vi "Frequ-sweep.vi"   [LabVIEW 2019]
uses:
  Global/Global Variables/global.vi
  Instrument_Setup.vi
  Global/Global Variables/Data_Display_global.vi
  Monitors/Utility/Monitor Communication/sub-vis/K6221_Open_Queue.vi
types:
  T1 = typedef "15T-Cluster.ctl" = cluster{"Magnet (T)":dbl, "Leads (T)":dbl, "Setpoint (T)":dbl, "Rate (T/min)":dbl, "Set":bool, "Zero":bool, "Hold":bool, "Go to zero":bool, "Go to Hold":bool, "Go to Set":bool, "Clamp":bool, "Switch Heater":bool, "Rate limit":bool, "Switch":bool, "Clamped":bool, "Persistent":bool, "Quenched":bool, "Sweeping":bool, "Select":bool}
  T2 = typedef "PSIO.ctl" = cluster{"Address":T3, "Version":enum16{"PS", "IPS"}}
  T3 = typedef "OxfordAddress.ctl" = cluster{"Com Port":i32, "ISOBUS Address":i32, "GPIB Address":i16, "Communication":enum16{"RS232", "ISOBUS", "GPIB", "Gateway"}}
  T4 = cluster{"Version\n":string, "Max Sweep":dbl[unit], "Max Field":dbl[unit], "IO Info":T2, "Switch htr dly":dbl[unit]}
  T5 = typedef "16T-Cluster.ctl" = cluster{"Clamp":bool, "Switch Heater":bool, "Go to Zero":bool, "Go to set":bool, "Go to Hold":bool, "Clamped":bool, "Quenched":bool, "Rate limit":bool, "Persistent":bool, "Hold":bool, "Set":bool, "Zero":bool, "Magnet (T)":dbl, "Leads (T)":dbl, "Magnet T (K)":dbl, "Switch":bool, "Setpoint (T)":dbl, "Rate (T/min)":dbl, "Select":bool, "Sweeping":bool}
  T6 = cluster{"Version\n":string, "Max Sweep(4.2K)":dbl[unit], "Max Sweep(2.2K)":dbl[unit], "Switch htr dly":dbl[unit], "Max Field(4.2K)":dbl[unit], "Max Field(2.2K)":dbl[unit], "Max lead res":dbl[unit], "IO Info":T2}
  T7 = typedef "K6221_Cluster.ctl" = cluster{"Plot Window":dbl[][], "A":dbl, "A (RMS)":dbl, "Hz":dbl, "I (A)":dbl, "f (Hz)":dbl, "Update":bool, "Offset":dbl, "Offset (A)":dbl, "Compliance":bool, "Output":bool, "Output Status":bool}
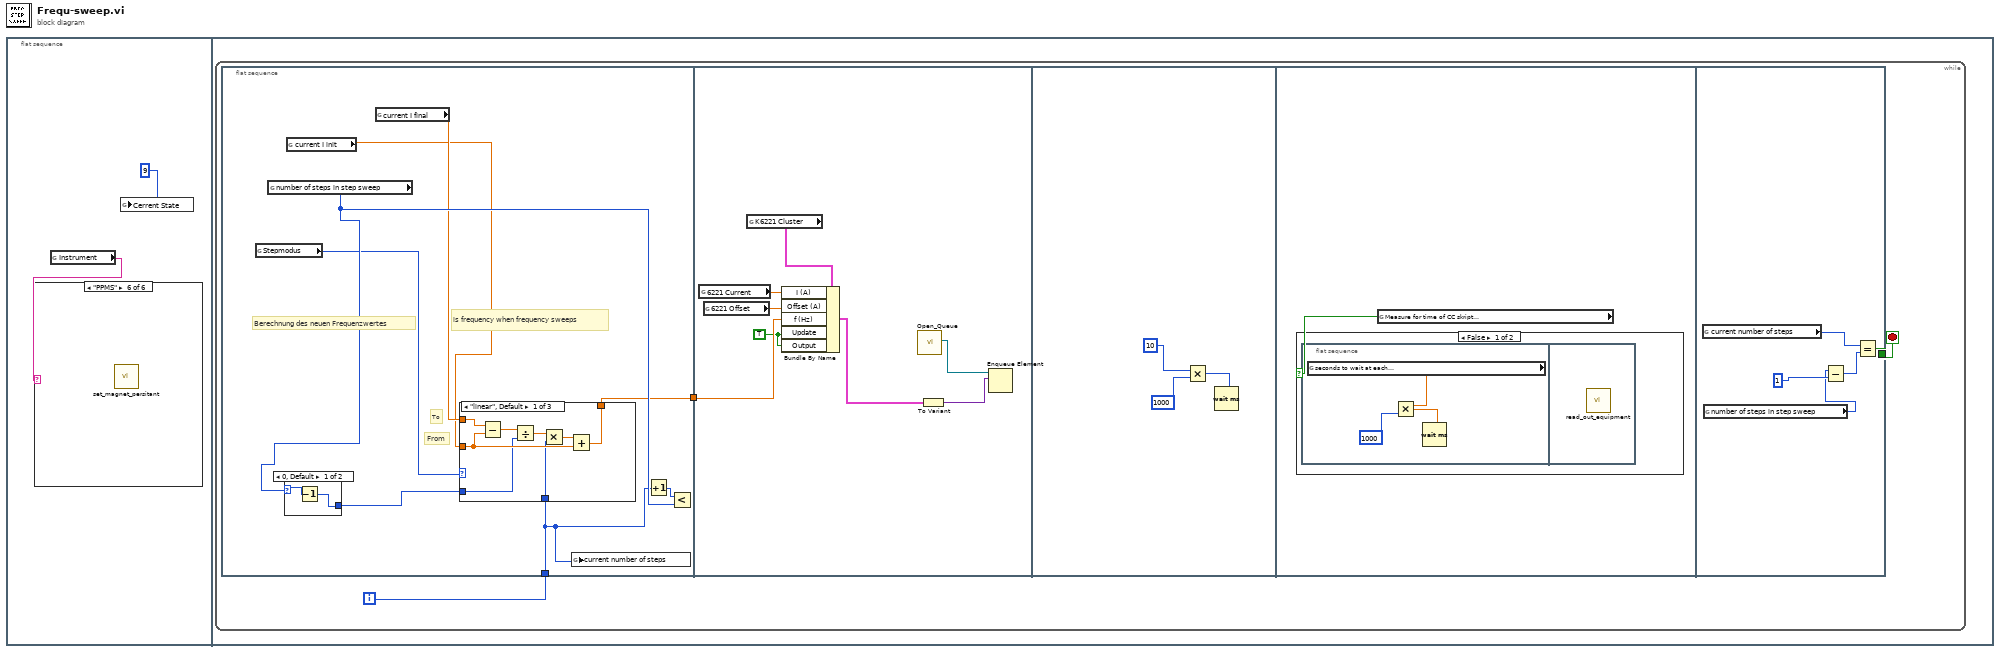
[diagram p0: block diagram]
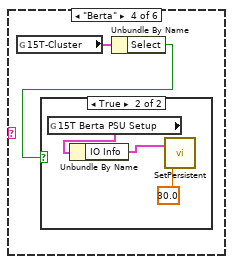
[diagram p5: hidden frame]
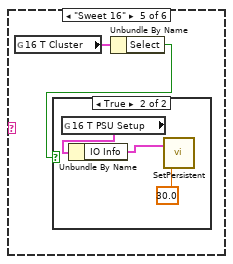
[diagram p7: hidden frame]
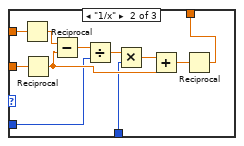
[diagram p10: hidden frame]
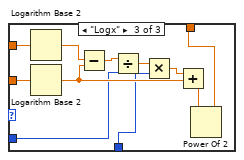
[diagram p11: hidden frame]
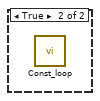
[diagram p12: hidden frame]
diagram:
  n1 = flat-sequence {
    frame #0 {
      n2 = global read "Instrument_Setup.vi" "Instrument"() -> (w1:string)
      n3 = case shown="\"PPMS\"" w1 {
        frame "AMI", Default {
        }
        frame "Mischer" {
        }
        frame "20T" {
        }
        frame "Berta" {
          n4 = global read "Data_Display_global.vi" "15T-Cluster"() -> (w4:T1)
          n5 = Unbundle By Name(w4) -> ("Select"=w3:bool)
          n6 = case shown="True" w3 {
            frame False {
            }
            frame True {
              n7 = global read "Instrument_Setup.vi" "15T Berta PSU Setup"() -> (w6:T4)
              n8 = Unbundle By Name(w6) -> ("IO Info"=w5:T2)
              n9 = call "SetPersistent.vi"("Switch Heater Dwell Time"=dbl[unit] 30.0, "IO Info"=w5) -> ()  [unwired: 1 in, 1 out]
            }
          }
        }
        frame "Sweet 16" {
          n10 = global read "Data_Display_global.vi" "16 T Cluster"() -> (w9:T5)
          n11 = Unbundle By Name(w9) -> ("Select"=w8:bool)
          n12 = case shown="True" w8 {
            frame False {
            }
            frame True {
              n13 = global read "Instrument_Setup.vi" "16 T PSU Setup"() -> (w11:T6)
              n14 = Unbundle By Name(w11) -> ("IO Info"=w10:T2)
              n15 = call "SetPersistent.vi"("Switch Heater Dwell Time"=dbl[unit] 30.0, "IO Info"=w10) -> ()  [unwired: 1 in, 1 out]
            }
          }
        }
        frame "PPMS" {
          n16 = call "set_magnet_persitant.vi"() -> ()  [unwired: 4 in]
        }
      }
      n17 = global write "global.vi" "Cerrent State"(9) -> ()
    }
    frame #1 {
      n18 = while {
        i -> [w14]
        stop <- w15 stop-if-true
        n19 = flat-sequence {
          tunnel: w14 -> [w17]
          tunnel: [w16] -> w13
          tunnel: w13 -> [w59]
          tunnel: [w75] -> w15
          frame #0 {
            # "From"
            # "To"
            # "is frequency when frequency sweeps"
            # "Berechnung des neuen Frequenzwertes"
            n20 = global read "Instrument_Setup.vi" "Stepmodus"() -> (w20:enum16{"linear", "1/x", "Logx"})
            n21 = global read "global.vi" "number of steps in step sweep"() -> (w21:i32)
            n22 = case shown="0, Default" w21 {
              selector: w21 -> [w25 w26]
              tunnel: [w24 w26] -> w22
              frame 0, Default {
                n23 = Decrement(x=w25) -> (x-1=w24:i32)
              }
              frame 1 {
              }
            }
            n24 = global read "global.vi" "current I init"() -> (w18:dbl)
            n25 = global read "global.vi" "current I final"() -> (w19:dbl)
            n26 = case shown="\"linear\", Default" w20 {
              tunnel: w19 -> [w34 w44 w56]
              tunnel: w18 -> [w31 w45 w55]
              tunnel: [w29 w39 w48] -> w16
              tunnel: w22 -> [w28 w36 w47]
              tunnel: w17 -> [w27 w35 w46]
              frame "linear", Default {
                n27 = Subtract(x=w34, y=w31) -> (x-y=w33:dbl)
                n28 = Divide(x=w33, y=w28) -> (x/y=w32:dbl)
                n29 = Multiply(x=w32, y=w27) -> (x*y=w30:dbl)
                n30 = Add(x=w30, y=w31) -> (x+y=w29:dbl)
              }
              frame "1/x" {
                n31 = Reciprocal(x=w44) -> (1/x=w38:dbl)
                n32 = Reciprocal(x=w45) -> (1/x=w37:dbl)
                n33 = Subtract(x=w38, y=w37) -> (x-y=w43:dbl)
                n34 = Divide(x=w43, y=w36) -> (x/y=w42:dbl)
                n35 = Multiply(x=w42, y=w35) -> (x*y=w41:dbl)
                n36 = Add(x=w41, y=w37) -> (x+y=w40:dbl)
                n37 = Reciprocal(x=w40) -> (1/x=w39:dbl)
              }
              frame "Logx" {
                n38 = Logarithm Base 2(1:w56) -> (0:w54:dbl)
                n39 = Logarithm Base 2(1:w55) -> (0:w50:dbl)
                n40 = Subtract(x=w54, y=w50) -> (x-y=w53:dbl)
                n41 = Divide(x=w53, y=w47) -> (x/y=w52:dbl)
                n42 = Multiply(x=w52, y=w46) -> (x*y=w51:dbl)
                n43 = Add(x=w51, y=w50) -> (x+y=w49:dbl)
                n44 = Power Of 2(x=w49) -> (2^x=w48:dbl)
              }
            }
            n45 = global write "Data_Display_global.vi" "current number of steps"(w17) -> ()
            n46 = Increment(x=w17) -> (x+1=w23:i32)
            n47 = Less?(x=w23, y=w21) -> ()  [unwired: 1 out]
          }
          frame #1 {
            w57 = TRUE
            n48 = global read "global.vi" "6221 Current"() -> (w61:dbl)
            n49 = global read "global.vi" "6221 Offset"() -> (w60:dbl)
            n50 = global read "Data_Display_global.vi" "K6221 Cluster"() -> (w64:T7)
            n51 = Bundle By Name(cluster=w64, "I (A)"=w61, "Offset (A)"=w60, "f (Hz)"=w59, "Update"=w57, "Output"=w57) -> (w63:T7)
            n52 = call-poly "Open_Queue.vi"() -> ("queue out"=w58:refnum<queue>)  [unwired: 10 in, 1 out]
            n53 = To Variant(anything=w63) -> (Variant=w62:variant)
            n54 = Enqueue Element(queue=w58, element=w62) -> ()  [unwired: 2 in, 3 out]
          }
          frame #2 {
            n55 = Multiply(x=10, y=u32 1000 ("milliseconds to wait")) -> (x*y=w66:u32)
            n56 = Wait (ms)(milliseconds to wait=w66) -> ()  [unwired: 1 out]
          }
          frame #3 {
            n57 = global read "Instrument_Setup.vi" "Measure for time of CC skript\nat each field step point"() -> (w68:bool)
            n58 = case shown="False" w68 {
              frame False {
                n59 = flat-sequence {
                  frame #0 {
                    n60 = global read "Instrument_Setup.vi" "seconds to wait at each\ncurrent step in a I-step sweep"() -> (w71:dbl)
                    n61 = Multiply(x=w71, y=u32 1000 ("milliseconds to wait")) -> (x*y=w69:dbl)
                    n62 = Wait (ms)(milliseconds to wait=w69) -> ()  [unwired: 1 out]
                  }
                  frame #1 {
                    n63 = call "read_out_equipment.vi"() -> ()  [unwired: 1 in]
                  }
                }
              }
              frame True {
                n64 = call "Const_loop.vi"() -> ()  [unwired: 4 in]
              }
            }
          }
          frame #4 {
            n65 = global read "Data_Display_global.vi" "current number of steps"() -> (w76:i32)
            n66 = global read "global.vi" "number of steps in step sweep"() -> (w73:i32)
            n67 = Subtract(x=w73, y=1) -> (x-y=w72:i32)
            n68 = Equal?(x=w76, y=w72) -> (x = y?=w75:bool)
          }
        }
      }
    }
  }
